vi "001 concatenació dos arrays.vi"() -> ()   [LabVIEW 2019]
panel:
  out "Frase 1 + 2":string
  in  "Frase 2":string
  in  "Frase":string
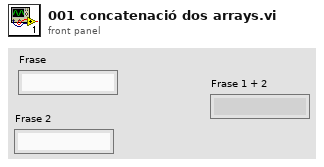
[diagram p1: front panel]
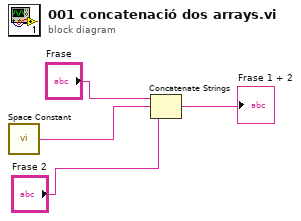
[diagram p0: block diagram]
diagram:
  n1 = call <vilib>:"Space Constant.vi"() -> ("String"=w1:string)
  n2 = Concatenate Strings("Frase", w1, "Frase 2") -> (→"Frase 1 + 2":string)
